vi "WCA_GET_HEAT_C.vi"(0 "Cartridge Band":u32=10, 1 "Slave Node in":cluster{"Address":i16, "Serial Number":i8[]}={"Address"=19, "Serial Number"=[16, 71, 55, 76, 1, 8, 0, -15]} {"Serial Number" format="%.0x"; "Address" format="%.0x"}, 2 "ObjHandle in":u32, 5 "POL":u32, 9 "avg":u32=1, 11 "error in (no error)":errorcluster) -> (4 "ObjHandle out":u32=92930112, 8 "get":dbl=0.35980224609375, 15 "error out":errorcluster)   [LabVIEW 2017]
uses:
  WCA_Global.vi
panel:
  # "Node Address"
  # "Serial Number"
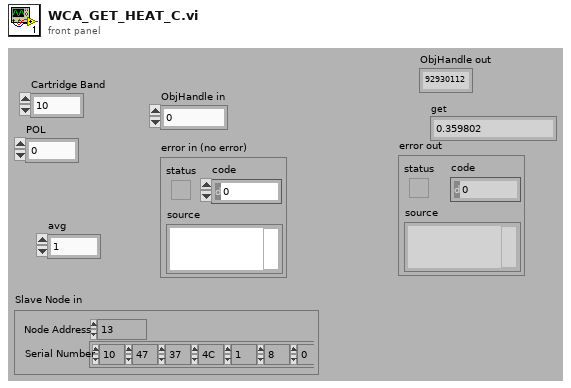
[diagram p1: front panel]
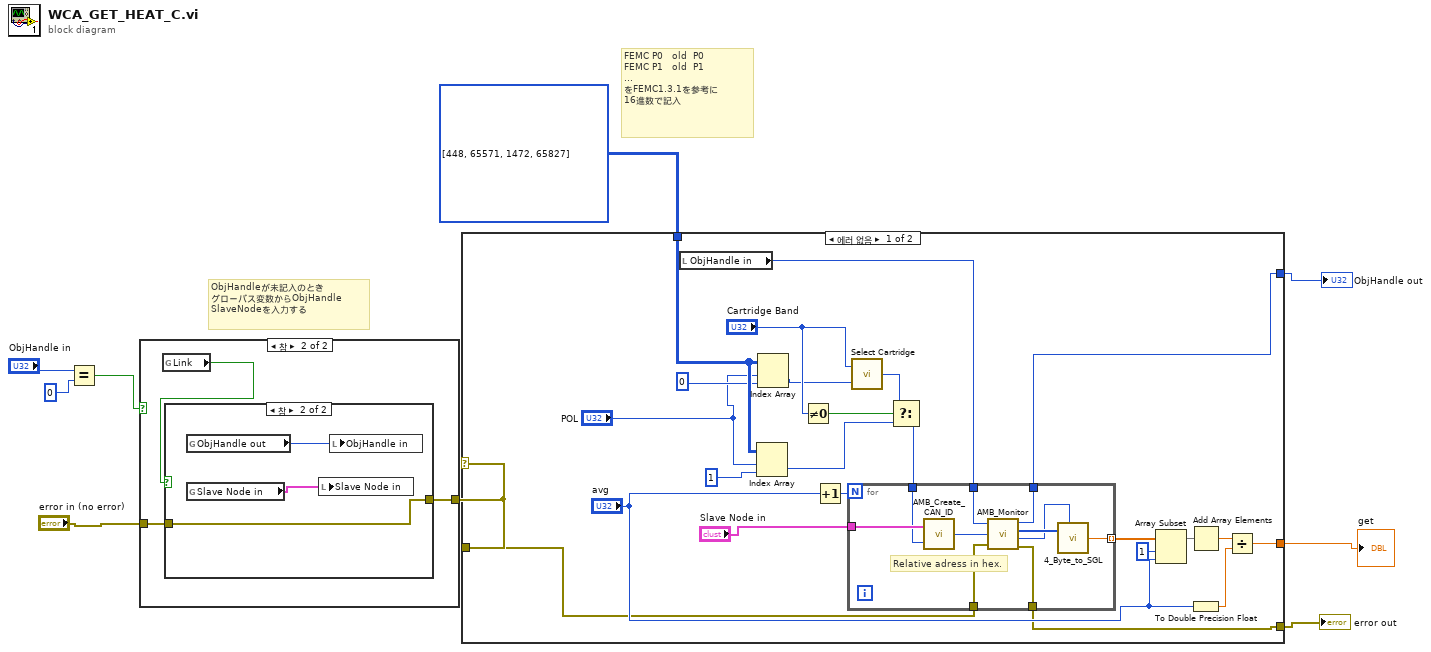
[diagram p0: block diagram]
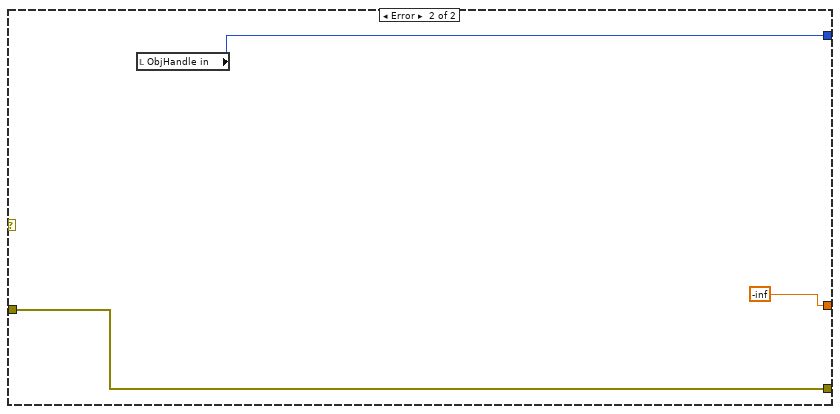
[diagram p2: hidden frame]
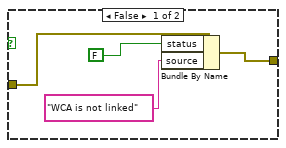
[diagram p4: hidden frame]
diagram:
  # "ObjHandleが未記入のとき\nグローバス変数からObjHandle\nSlaveNodeを入力する"
  # "FEMC P0   old  P0\nFEMC P1   old  P1\n...\nをFEMC1.3.1を参考に\n16進数で記入"
  n1 = Equal?(x="ObjHandle in", y=0) -> (x = y?=w7:bool)
  n2 = case shown="참" w7 {
    tunnel: "error in (no error)" -> [w10 w13]
    tunnel: [w10 w12] -> w5
    frame False {
    }
    frame True {
      n3 = global read "WCA_Global.vi" "Link"() -> (w11:bool)
      n4 = case shown="참" w11 {
        tunnel: w13 -> [w17 w18]
        tunnel: [w14 w18] -> w12
        frame False {
          n5 = Bundle By Name(cluster=w17, "status"=FALSE, "source"="WCA is not linked") -> (w14:errorcluster)
        }
        frame True {
          n6 = global read "WCA_Global.vi" "ObjHandle out"() -> (w20:u32)
          n7 = global read "WCA_Global.vi" "Slave Node in"() -> (w19:cluster{"Address":i16, "Serial Number":i8[]})
          n8 = local write "Slave Node in"(w19) -> ()
          n9 = local write "ObjHandle in"(w20) -> ()
        }
      }
    }
  }
  n10 = case shown="에러 없음" w5 {
    tunnel: w5 -> [w30 w56]
    tunnel: [w27 w55] -> w4
    tunnel: [w29 w56] -> w3
    tunnel: i32[][] [[448, 65571], [1472, 65827]] -> [w43 _]
    tunnel: [w33 -inf] -> w1
    frame No Error {
      n11 = local read "ObjHandle in"() -> (w28:u32)
      n12 = Index Array(array=w43, index (row)="POL", index (col)=1) -> (element=w25:i32)
      n13 = Index Array(array=w43, index (row)="POL", index (col)=0) -> (element=w24:i32)
      n14 = Not Equal To 0?(x="Cartridge Band") -> (x != 0?=w38:bool)
      n15 = Increment(x="avg") -> (x+1=w41:u32)
      n16 = call "Select Cartridge.vi"("Relative Address in"=w24, "Cartridge band"="Cartridge Band") -> ("Relative Address out"=w39:u32)
      n17 = Select(t=w39, s=w38, f=w25) -> (s? t:f=w40:u32)
      n18 = for {
        N: w41 -> [_]
        tunnel: w28 -> [w52]
        tunnel: [w51] -> w27
        tunnel: [w50] -> w29
        tunnel: w30 -> [w49]
        tunnel: "Slave Node in" -> [w48]
        tunnel: [w46] -> w37 mode=indexing
        tunnel: w40 -> [w44]
        # "Relative adress in hex."
        n19 = call "AMB_Create_CAN_ID.vi"("Relative Address in"=w44, "Slave Node in"=w48) -> ("CAN ID out"=w53:u32)
        n20 = call "AMB_Monitor.vi"("ObjHandle in"=w52, "CAN ID in"=w53, "error in"=w49) -> ("ObjHandle out"=w51:u32, "Data Array out"=w47:u8[], "Data Length out"=w45:u8, "error out"=w50:errorcluster)
        n21 = call "4_Byte_to_SGL.vi"("Array of 4 bytes"=w47, "number of valid bytes"=w45) -> ("Number"=w46:sgl)  [unwired: 1 out]
      }
      n22 = Array Subset(array=w37, index=1, length="avg") -> (w35:sgl[])
      n23 = Add Array Elements(numeric array=w35) -> (sum=w34:sgl)
      n24 = To Double Precision Float(number="avg") -> (double precision float=w42:dbl)
      n25 = Divide(x=w34, y=w42) -> (x/y=w33:dbl)
    }
    frame Error {
      n26 = local read "ObjHandle in"() -> (w55:u32)
    }
  }
  "ObjHandle out" <- w4
  "error out" <- w3
  "get" <- w1
